vi "Coding_morse2.vi"() -> ()   [LabVIEW 2022 SP3]
panel:
  out "String":string
  out "Current code":string
  out "Wait time between words":dbl
  out "Waiting until next word":bool
  in  "Dit time(ms)":dbl
  out "current dit/dash time":dbl
  out "Character code remained":i32
  in  "Frequency":dbl=500.0
  in  "Volume":dbl(knob) scale=0.0..100.0
  out "Whole code":string[](array[string])
  in  "Input Words words":string
  in  "stop":bool
  in  "Alphabet":string[][](array[string])=[["a", ".-"], ["b", "-..."], ["c", "-.-."], ["d", "-.."], ["e", "."], ["f", "..-."], ["g", "--."], ["h", "...."], ["i", ".."], ["j", ".---"], ["k", "-.-"], ["l", ".-.."], ["m", "--"], ["n", "-."], ["o", "---"], ["p", ".--."], ["q", "--.-"], ["r", ".-."], ["s", "..."], ["t", "-"], ["u", "..-"], ["v", "...-"], ["w", ".--"], ["x", "-..-"], ["y", "-.--"], ["z", "--.."], ["1", ".----"], ["2", "..---"], ["3", "...--"], ["4", "....-"], ["5", "....."], ["6", "-...."], ["7", "--..."], ["8", "---.."], ["9", "----."], ["0", "-----"], [" ", "space"]]
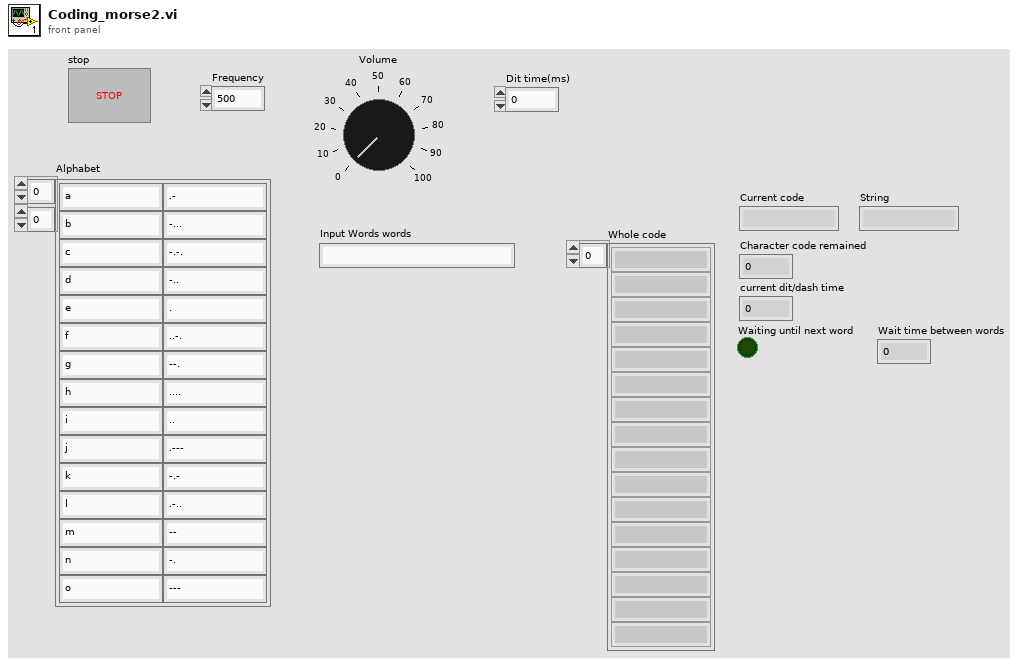
[diagram p1: front panel]
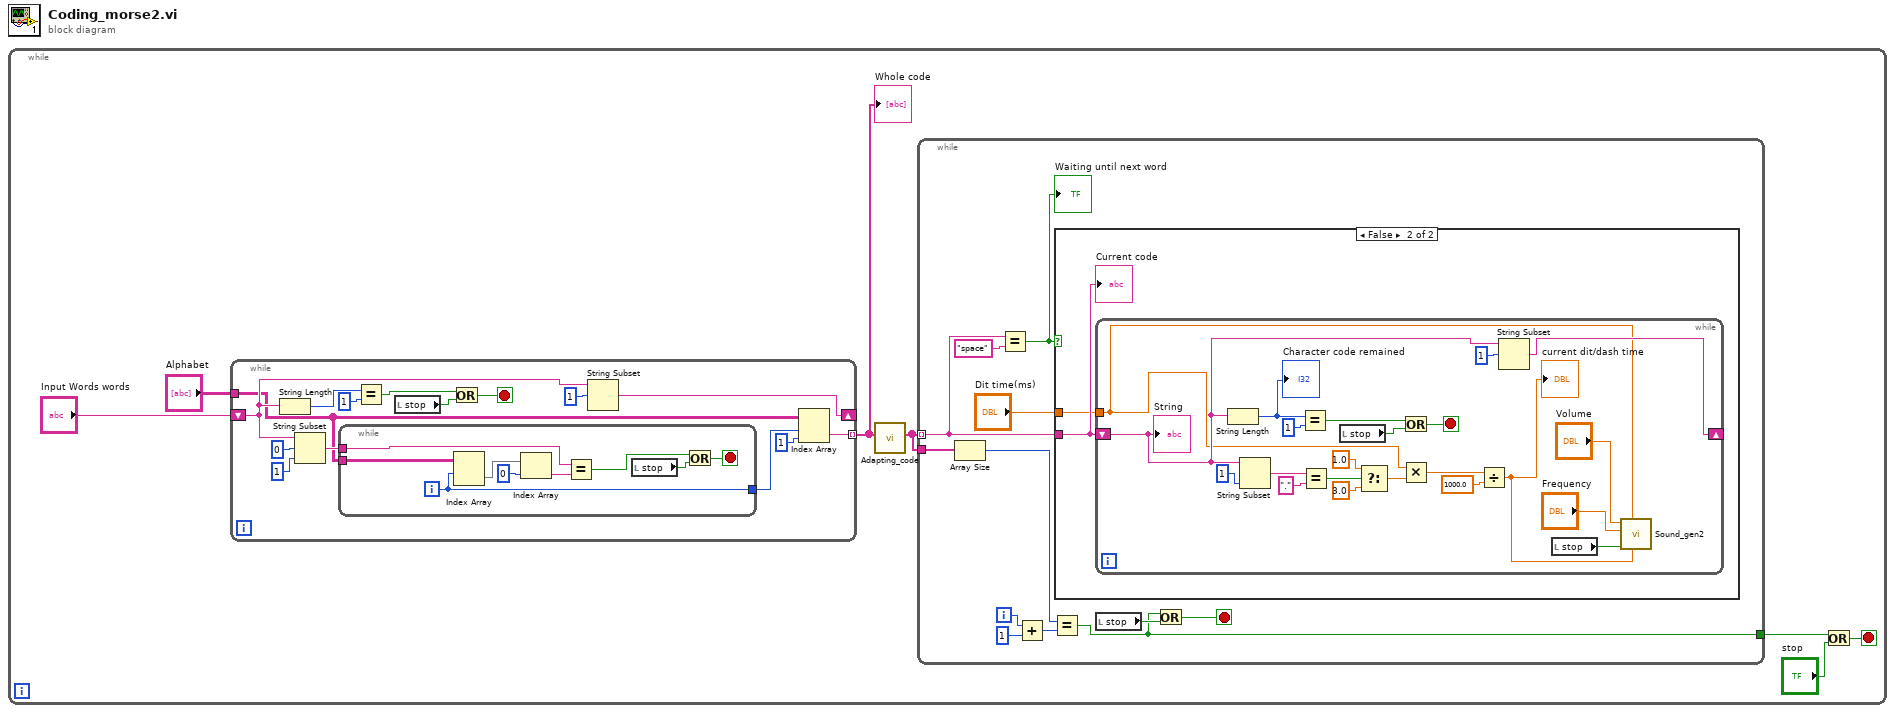
[diagram p0: block diagram]
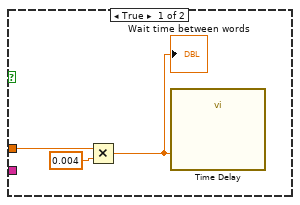
[diagram p2: hidden frame]
diagram:
  n1 = while {
    stop <- w3 stop-if-true
    n2 = while {
      shift-right: [w55] -> _
      shift-left: "Input Words words" -> [w56]
      tunnel: "Alphabet" -> [w52]
      tunnel: [w47] -> w2 mode=indexing
      stop <- w48 stop-if-true
      n3 = String Length(string=w56) -> (length=w49:i32)
      n4 = String Subset(string=w56, offset (0)=0, length (rest)=1 ("length (rest)")) -> (substring=w53:string)
      n5 = while {
        tunnel: w52 -> [w70]
        tunnel: w53 -> [w67]
        tunnel: [w62] -> w51
        i -> [w62]
        stop <- w63 stop-if-true
        n6 = Index Array(array=w70, index (row)=w62) -> (element=w68:string[])  [unwired: 1 in]
        n7 = Index Array(array=w68, index=0) -> (element=w66:string)
        n8 = Equal?(x=w67, y=w66) -> (x = y?=w65:bool)
        n9 = local read "stop"() -> (w64:bool)
        n10 = Or(x=w65, y=w64) -> (x .or. y?=w63:bool)
      }
      n11 = Equal?(x=w49, y=1) -> (x = y?=w59:bool)
      n12 = local read "stop"() -> (w60:bool)
      n13 = Or(x=w59, y=w60) -> (x .or. y?=w48:bool)
      n14 = String Subset(string=w56, offset (0)=1) -> (substring=w55:string)  [unwired: 1 in]
      n15 = Index Array(array=w52, index (row)=w51, index (col)=1 ("disabled index (col)")) -> (element=w47:string)
    }
    "Whole code" <- w2
    n16 = call "Adapting_code.vi"("Code"=w2) -> ("Code with an extra dot"=w1:string[])  [unwired: 10 in]
    n17 = while {
      tunnel: w1 -> [w10] mode=indexing
      tunnel: w1 -> [w16]
      tunnel: [w18] -> w5
      i -> [w14]
      stop <- w17 stop-if-true
      n18 = Array Size(array=w16) -> (size(s)=w15:i32)
      n19 = Equal?(x=w10, y="space") -> (x = y?=w8:bool)
      "Waiting until next word" <- w8
      n20 = Add(x=w14, y=1) -> (x+y=w12:i32)
      n21 = Equal?(x=w15, y=w12) -> (x = y?=w18:bool)
      n22 = case shown="False" w8 {
        tunnel: w10 -> [_ w24]
        tunnel: "Dit time(ms)" -> [w21 w23]
        frame True {
          n23 = Multiply(x=w21, y=0.004) -> (x*y=w20:dbl)
          "Wait time between words" <- w20
          n24 = call "Time Delay"("Delay Time (s)"=w20) -> ()  [unwired: 10 in, 1 out]
        }
        frame False {
          n25 = while {
            shift-right: [w28] -> _
            shift-left: w24 -> [w30]
            tunnel: w23 -> [w25]
            stop <- w44 stop-if-true
            n26 = String Length(string=w30) -> (length=w46:i32)
            "Character code remained" <- w46
            n27 = String Subset(string=w30, length (rest)=1 ("length (rest)")) -> (substring=w41:string)  [unwired: 1 in]
            n28 = Equal?(x=w46, y=1) -> (x = y?=w45:bool)
            n29 = Equal?(x=w41, y=".") -> (x = y?=w40:bool)
            n30 = local read "stop"() -> (w43:bool)
            n31 = Select(t=1.0, s=w40, f=3.0) -> (s? t:f=w42:dbl)
            n32 = Or(x=w45, y=w43) -> (x .or. y?=w44:bool)
            n33 = Multiply(x=w25, y=w42) -> (x*y=w33:dbl)
            n34 = Divide(x=w33, y=1000.0) -> (x/y=w27:dbl)
            "current dit/dash time" <- w27
            n35 = String Subset(string=w30, offset (0)=1) -> (substring=w28:string)  [unwired: 1 in]
            n36 = local read "stop"() -> (w26:bool)
            n37 = call "Sound_gen2.vi"("Sound time(s)"=w27, "Dit time(ms)"=w25, "stop"=w26, "Frequency"="Frequency", "Volume"="Volume") -> ()  [unwired: 6 in, 1 out]
            "String" <- w30
          }
          "Current code" <- w24
        }
      }
      n38 = local read "stop"() -> (w19:bool)
      n39 = Or(x=w18, y=w19) -> (x .or. y?=w17:bool)
    }
    n40 = Or(x=w5, y="stop") -> (x .or. y?=w3:bool)
  }
